vi "UsrProfiles-Rename profile.vi"   [LabVIEW 2020]
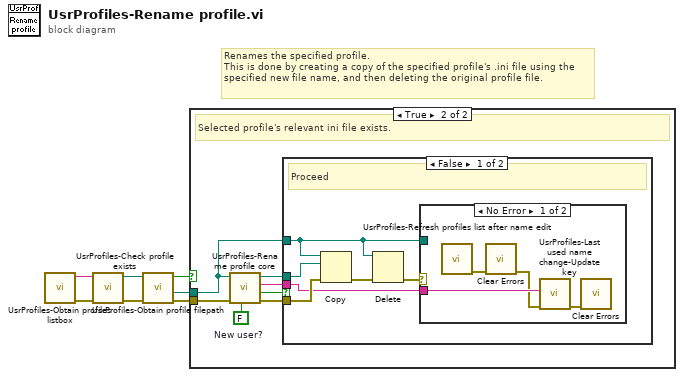
[diagram p0: block diagram]
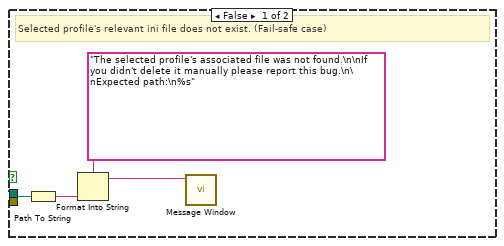
[diagram p2: hidden frame]
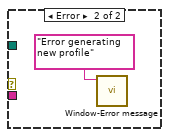
[diagram p3: hidden frame]
diagram:
  # "Renames the specified profile.\nThis is done by creating a copy of the specified profile's .ini file using the specified new file name, and then deleting the original profile file."
  n1 = call "UsrProfiles-Obtain profiles listbox.vi"() -> ("error out"=w6:errorcluster, "Selected profile's name"=w7:string)  [unwired: 8 in, 2 out]
  n2 = call "UsrProfiles-Obtain profile filepath.vi"("error in"=w6, "Profile name"=w7) -> ("error out"=w5:errorcluster, "Profile filepath"=w1:path)  [unwired: 8 in]
  n3 = call "UsrProfiles-Check profile exists.vi"("error in"=w5, "Profile file path"=w1) -> ("error out"=w4:errorcluster, "Profile's file path"=w3:path, "Profile file exists"=w2:bool)  [unwired: 7 in]
  n4 = case shown="True" w2 {
    tunnel: w4 -> [_ w13]
    tunnel: w3 -> [w11 w16]
    frame False {
      # "Selected profile's relevant ini file does not exist. (Fail-safe case)"
      n5 = Path To String(path=w11) -> (string=w10:string)
      n6 = Format Into String(format string="The selected profile's associated file was not found.\n\nIf you didn't delete it manually please report this bug.\n\nExpected path:\n%s", w10) -> (resulting string=w8:string)  [unwired: 2 in, 1 out]
      n7 = call "Message Window.vi"("Message string"=w8) -> ()  [unwired: 10 in, 1 out]
    }
    frame True {
      w17 = FALSE  # New user?
      # "Selected profile's relevant ini file exists."
      n8 = call "UsrProfiles-Rename profile core.vi"("New user"=w17, "error in (no error)"=w13, "Source profile's filepath"=w16) -> ("error out"=w14:errorcluster, "Cancelled"=w15:bool, "New profile name"=w12:string, "Filepath of profile to be created"=w18:path)  [unwired: 5 in]
      n9 = case shown="False" w15 {
        tunnel: w18 -> [w20 _]
        tunnel: w14 -> [w24 _]
        tunnel: w16 -> [w21 _]
        tunnel: w12 -> [w19 _]
        frame False {
          # "Proceed"
          n10 = Copy(8:w24, 10:w20, 11:w21) -> (0:w23:errorcluster)  [unwired: 2 in, 2 out]
          n11 = Delete(path (use dialog)=w21, error in=w23) -> (error out=w22:errorcluster)  [unwired: 3 in, 2 out]
          n12 = case shown="No Error" w22 {
            tunnel: w21 -> [_ _]
            tunnel: w19 -> [w27 _]
            frame No Error {
              n13 = call "UsrProfiles-Refresh profiles list after name edit.vi"() -> ("error out"=w28:errorcluster)  [unwired: 11 in]
              n14 = call <vilib>:"Clear Errors.vi"("error in (no error)"=w28) -> ("error out"=w25:errorcluster)  [unwired: 5 in, 1 out]
              n15 = call "UsrProfiles-Last used name change-Update key.vi"("error in (no error)"=w25, "Modified profile name"=w27) -> ("error out"=w26:errorcluster)  [unwired: 9 in]
              n16 = call <vilib>:"Clear Errors.vi"("error in (no error)"=w26) -> ()  [unwired: 5 in, 2 out]
            }
            frame Error {
              n17 = call "Window-Error message.vi"("Message"="Error generating new profile") -> ()  [unwired: 10 in, 1 out]
            }
          }
        }
        frame True {
          # "Cancelled"
        }
      }
    }
  }
